vi "Start Data Capture.vi"(8 "Error In":errorcluster, 9 "ADC Type in":T1={"Channels"="", "Range"=0.0, "Resolution"=2.0, "Sampling Rate"=0.0}, 10 "Start/Stop in":bool, 11 "Model in":refnum<class "Model.lvclass">) -> (0 "Error Out":errorcluster, 3 "Model out":refnum<class "Model.lvclass">)   [LabVIEW 2021, in "Model.lvclass"]
doc: "This VI sends the Adc type specifications data to the analog to digital convertor VI."
uses:
  Model.lvclass
  Controls/Queue Operation.ctl
  Controls/State Cluster.ctl
  Controls/ADC Type.ctl
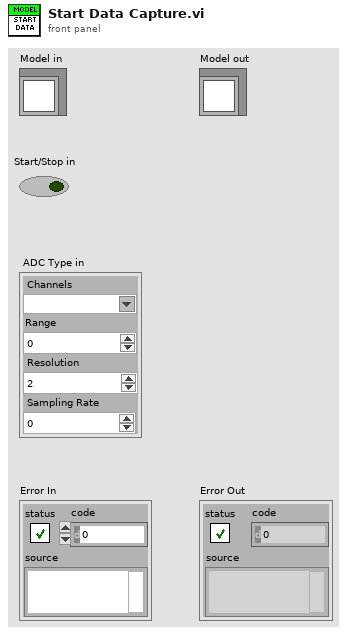
[diagram p1: front panel]
types:
  T1 = typedef "ADC Type.ctl" = cluster{"Channels":string, "Range":dbl, "Resolution":dbl, "Sampling Rate":dbl}
  T2 = typedef "State Cluster.ctl" = cluster{"State":string, "Data":variant}
  T3 = typedef "Queue Operation.ctl" = enum16{"Create", "Enqueue", "Enqueue N", "Enstack", "Dequeue", "Flush", "Release"}
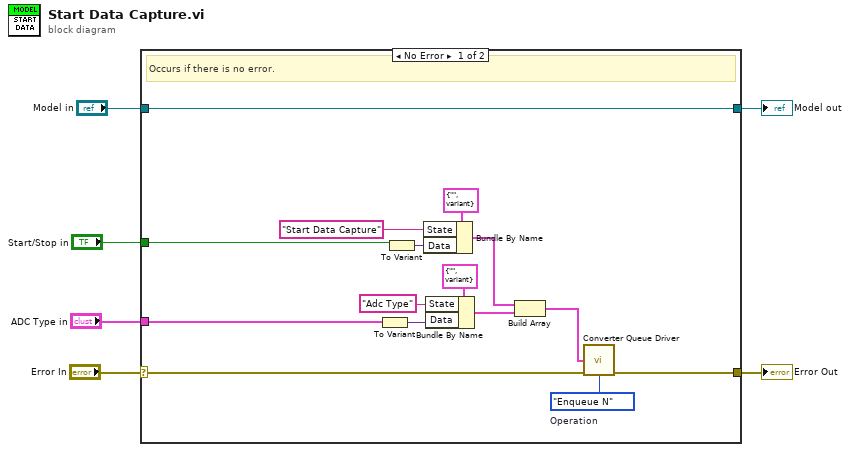
[diagram p0: block diagram]
diagram:
  n1 = case shown="No Error" "Error In" {
    selector: "Error In" -> [w11 w23]
    tunnel: [w10 w23] -> w5
    tunnel: [w21 w22] -> w3
    tunnel: "Model in" -> [w21 w22]
    tunnel: "Start/Stop in" -> [w9 _]
    tunnel: "ADC Type in" -> [w8 _]
    frame No Error {
      w20 = Queue_Operation."Enqueue N"  # Operation
      # "Occurs if there is no error."
      n2 = To Variant(anything=w8) -> (Variant=w15:variant)
      n3 = To Variant(anything=w9) -> (Variant=w17:variant)
      n4 = Bundle By Name(cluster=T2 {"State"="", "Data"=variant} ("State"), "State"="Start Data Capture", "Data"=w17) -> (w14:T2)
      n5 = Bundle By Name(cluster=T2 {"State"="", "Data"=variant} ("State"), "State"="Adc Type", "Data"=w15) -> (w13:T2)
      n6 = Build Array(w14, w13) -> (w12:T2[])
      n7 = call "Converter Queue Driver.vi"("States[]"=w12, "error in (no error)"=w11, "Operation"=w20) -> ("error out"=w10:errorcluster)  [unwired: 11 in, 1 out]
    }
    frame Error {
      # "Occurs if there is any error."
    }
  }
  "Error Out" <- w5
  "Model out" <- w3
